vi "ExOpenGlobalPulser64.vi"(0 "error in (no error)":errorcluster) -> (1 "Pulser Handle":u32, 2 "error out":errorcluster)   [LabVIEW 2010]
uses:
  CamHandle.vi
  PulserHandle.vi
panel:
  out "Pulser open":bool
  # "ExPulser:\nThis opens a PTG object."
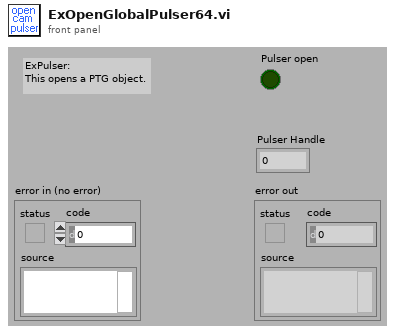
[diagram p1: front panel]
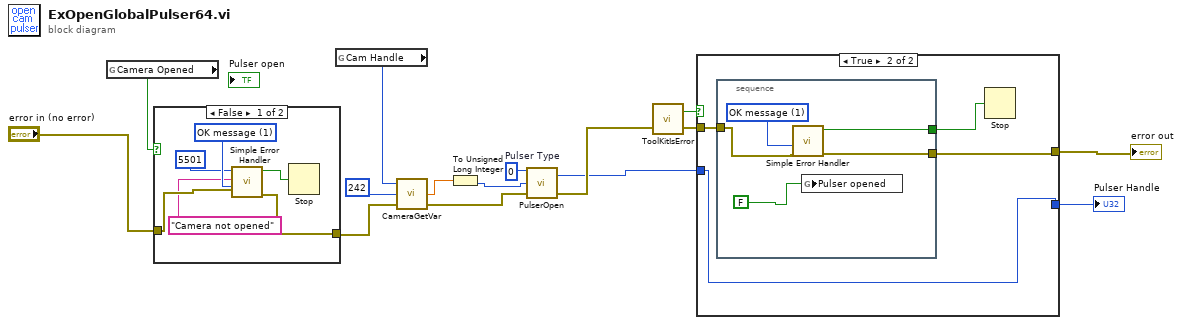
[diagram p0: block diagram]
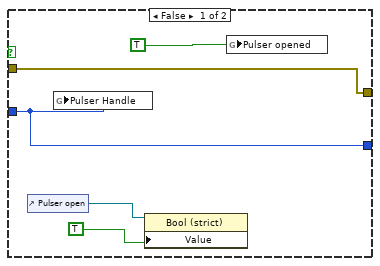
[diagram p2: hidden frame]
diagram:
  w15 = u32 0  # Pulser Type
  n1 = global read "CamHandle.vi" "Camera Opened"() -> (w14:bool)
  n2 = case shown="False" w14 {
    tunnel: "error in (no error)" -> [w20 w22]
    tunnel: [w19 w22] -> w4
    frame False {
      w21 = u16 1 items=["no dialog", "OK message", "continue or stop message"] ("type of dialog (OK msg:1)")
      n3 = call <vilib>:"Simple Error Handler.vi"("error code (no error:0)"=5501, "error source (\" \")"="Camera not opened", "type of dialog (OK msg:1)"=w21, "error in (no error)"=w20) -> ("error?"=w17:bool, "error out"=w19:errorcluster)  [unwired: 1 in, 3 out]
      n4 = Stop(stop? (T)=w17) -> ()
    }
    frame True {
    }
  }
  n5 = global read "CamHandle.vi" "Cam Handle"() -> (w5:u32)
  n6 = call <userlib>:"CameraGetVar.vi"("error in"=w4, "Parameter ID"=242, "Camera Handle"=w5) -> ("error out"=w3:errorcluster, "Value"=w2:dbl)  [unwired: 1 out]
  n7 = To Unsigned Long Integer(number=w2) -> (unsigned 32bit integer=w1:u32)
  n8 = call <userlib>:"PulserOpen.vi"("error in"=w3, "Camera Handle"=w1, "Pulser Type"=w15) -> ("error out"=w12:errorcluster, "Pulser Handle"=w9:u32)
  n9 = call <userlib>:"ToolKitIsError.vi"("error in"=w12) -> ("error out"=w10:errorcluster, "Error Flag"=w11:bool)  [unwired: 1 in]
  n10 = case shown="True" w11 {
    tunnel: w10 -> [w24 w31]
    tunnel: [w24 w30] -> w8
    tunnel: w9 -> [w23 w28]
    tunnel: [w23 w28] -> w7
    frame False {
      n11 = control-ref of="Pulser open"() -> (w26:refnum<vi>)
      n12 = global write "PulserHandle.vi" "Pulser Handle"(w23) -> ()
      n13 = property class="Bool (strict)"(reference=w26, "Value"=TRUE) -> ()  [unwired: 1 in, 2 out]
      n14 = global write "PulserHandle.vi" "Pulser opened"(TRUE) -> ()
    }
    frame True {
      n15 = stacked-sequence {
        tunnel: w31 -> [w35]
        tunnel: [w34] -> w29
        tunnel: [w33] -> w30
        frame #0 {
          w36 = u16 1 items=["no dialog", "OK message", "continue or stop message"] ("type of dialog (OK msg:1)")
          n16 = call <vilib>:"Simple Error Handler.vi"("type of dialog (OK msg:1)"=w36, "error in (no error)"=w35) -> ("error?"=w34:bool, "error out"=w33:errorcluster)  [unwired: 3 in, 3 out]
          n17 = global write "PulserHandle.vi" "Pulser opened"(FALSE) -> ()
        }
      }
      n18 = Stop(stop? (T)=w29) -> ()
    }
  }
  "error out" <- w8
  "Pulser Handle" <- w7
